vi "Finish.vi"() -> ()   [LabVIEW 2016]
doc: "This VI is called just before exiting. It is expected to close I/O refnum, save collected data, etc."
uses:
  Robot Global Data.vi
panel:
  out "Extra Elements":i32
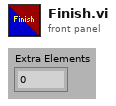
[diagram p1: front panel]
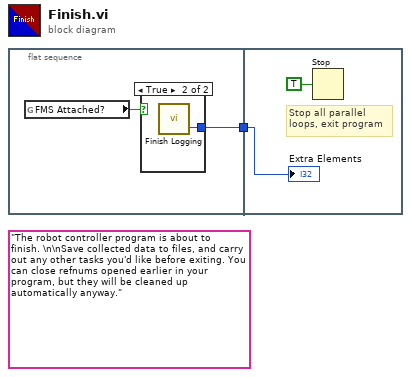
[diagram p0: block diagram]
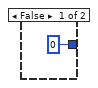
[diagram p2: hidden frame]
diagram:
  (unwired) "The robot controller program is about to finish. \n\nSave collected data to files, and carry out any other tasks you'd like before exiting. You can close refnums opened earlier in your program, but they will be cleaned up automatically anyway."
  n1 = flat-sequence {
    tunnel: [w2] -> w1
    tunnel: w1 -> [w6]
    frame #0 {
      n2 = global read "Robot Global Data.vi" "FMS Attached?"() -> (w3:bool)
      n3 = case shown="True" w3 {
        tunnel: [0 ("Extra Elements") w5] -> w2
        frame False {
        }
        frame True {
          n4 = call "Finish Logging.vi"() -> ("Extra Elements"=w5:i32)  [unwired: 1 in, 1 out]
        }
      }
    }
    frame #1 {
      # "Stop all parallel\nloops, exit program"
      n5 = Stop(stop? (T)=TRUE ("Quit")) -> ()
      "Extra Elements" <- w6
    }
  }
